vi "ACT Control.vi"() -> ()   [LabVIEW 2022 SP3, in "BC79.lvclass"]
uses:
  BC79.lvclass
  BC79.lvclass/BC79.ctl
  MD_modules/MD420/MD420.lvclass
panel:
  in  "MD420.lvclass":refnum<class "MD420.lvclass">
  in  "error in":errorcluster
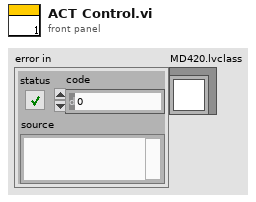
[diagram p1: front panel]
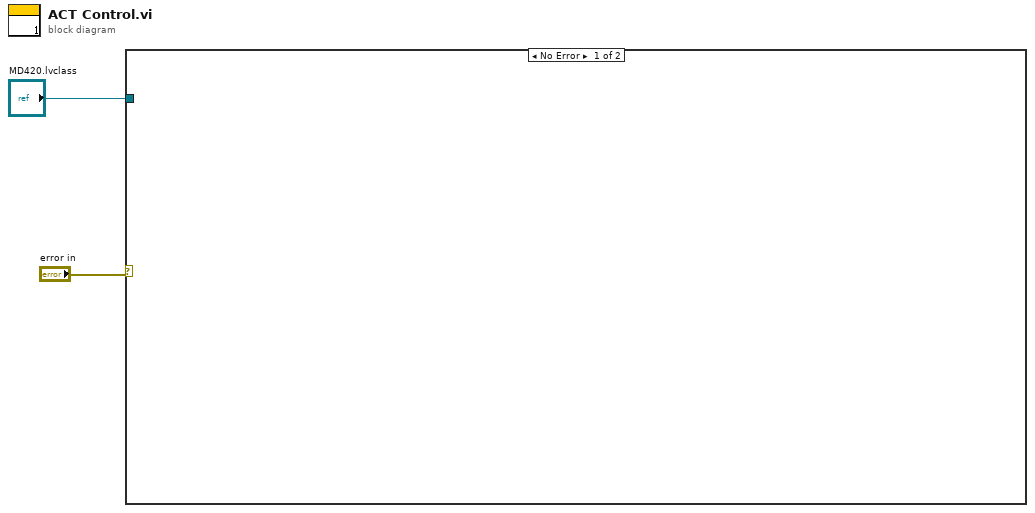
[diagram p0: block diagram]
diagram:
  n1 = case shown="No Error" "error in" {
    tunnel: "MD420.lvclass" -> [_ _]
    frame No Error {
    }
    frame Error {
    }
  }
